vi "Equals.vi"(1 "comparable b":dbl, 2 "comparable a":dbl, 3 "Equals Functor":refnum<class "Equal With Epsilon Functor.lvclass">) -> (0 "equal?":bool)   [LabVIEW 2019, in "Equal With Epsilon Functor.lvclass"]
doc: "Returns whether <b>comparable a</b> is equal to <b>comparable b</b> within some given distance <b>epsilon</b>, defined by the class. If epsilon has never been assigned, this VI uses the <b>Machine Epsilon</b> constant value."
uses:
  Equal With Epsilon Functor.lvclass
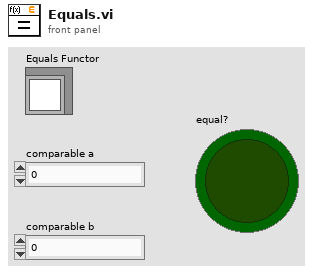
[diagram p1: front panel]
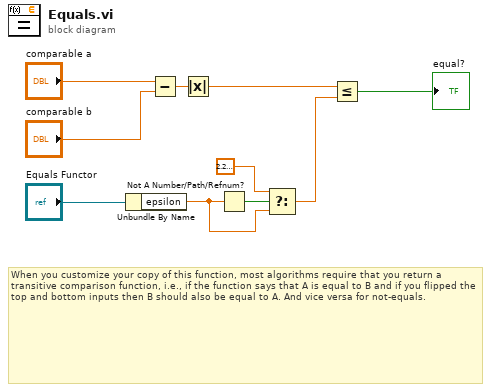
[diagram p0: block diagram]
diagram:
  # "When you customize your copy of this function, most algorithms require that you return a transitive comparison function, i.e., if the function says that A is equal to B and if you flipped the top and bottom inputs then B should also be equal to A. And vice versa for not-equals."
  n1 = Unbundle By Name("Equals Functor") -> ("epsilon"=w2:dbl)
  n2 = Subtract(x="comparable a", y="comparable b") -> (x-y=w7:dbl)
  n3 = Absolute Value(x=w7) -> (abs(x)=w6:dbl)
  n4 = Not A Number/Path/Refnum?(number/path/refnum=w2) -> (NaN/Path/Refnum?=w4:bool)
  n5 = Select(t=2.220446049250313e-16, s=w4, f=w2) -> (s? t:f=w1:dbl)
  n6 = Less Or Equal?(x=w6, y=w1) -> (x <= y?=→"equal?":bool)
